vi "Pose3d_Div.vi"(9 "Scalar":dbl, 11 "in Pose3d":T1={"Translation3d"={"X"=0.0, "Y"=0.0, "Z"=0.0}, "Rotation3d"={"Q_quaternion"={"R"=1.0, "V"=[0.0, 0.0, 0.0]}}} {"Translation3d"."Z" format="%14.3f"; "Translation3d"."Y" format="%14.3f"; "Translation3d"."X" format="%14.3f"}) -> (3 "out Pose3d":T1={"Translation3d"={"X"=0.0, "Y"=0.0, "Z"=0.0}, "Rotation3d"={"Q_quaternion"={"R"=1.0, "V"=[0.0, 0.0, 0.0]}}} {"Translation3d"."Z" format="%14.3f"; "Translation3d"."Y" format="%14.3f"; "Translation3d"."X" format="%14.3f"})   [LabVIEW 2019, in "Trajectory_Library.lvlib"]
doc: "Divide the pose by the given scalar and returns the new pose3d. \n\nParameters:\n - IN POSE3D - The input POSE data structure\n - Scalar - The value to divide the pose by.\n\nReturn:\n - OUT POSE3D - The output pose."
uses:
  TypeDef/POSE3D.ctl
  TypeDef/TRANSLATION3D.ctl
  TypeDef/ROTATION3D.ctl
  TypeDef/QUATERNION.ctl
  Translation3d_Create.vi
  Translation3d_GetXYZ.vi
  Rotation3d_Create_AxisAngle.vi
  Rotation3d_GetQuaterion.vi
  Quaternion_Get_Vect.vi
  Quaternion_Get_W.vi
  Quaternion_New.vi
  Rotation3d_Create_Default.vi
  Vector_Norm.vi
  VecBuilder_ArrayBy1Fill.vi
  Quaternion_New_Default.vi
  MatBuilder_Create.vi
  Trajectory_Library.lvlib
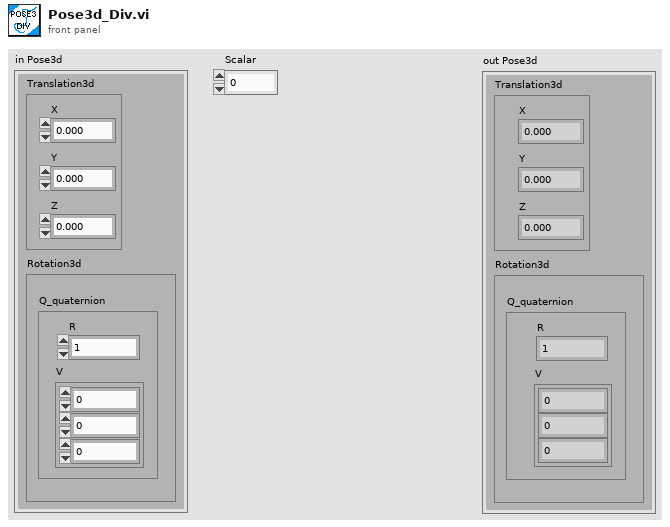
[diagram p1: front panel]
types:
  T1 = typedef "Trajectory_Library.lvlib/POSE3D.ctl" = cluster{"Translation3d":T2, "Rotation3d":T3}
  T2 = typedef "Trajectory_Library.lvlib/TRANSLATION3D.ctl" = cluster{"X":dbl, "Y":dbl, "Z":dbl}
  T3 = typedef "Trajectory_Library.lvlib/ROTATION3D.ctl" = cluster{"Q_quaternion":T4}
  T4 = typedef "Trajectory_Library.lvlib/QUATERNION.ctl" = cluster{"R":dbl, "V":dbl[]}
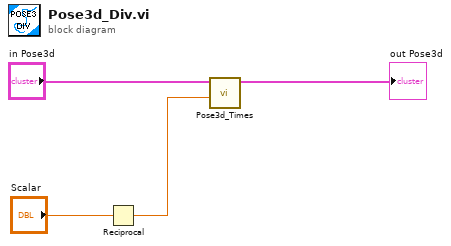
[diagram p0: block diagram]
diagram:
  n1 = Reciprocal(x="Scalar") -> (1/x=w3:dbl)
  n2 = call "Pose3d_Times.vi"("Scalar"=w3, "in Pose3d"="in Pose3d") -> ("out Pose3d"=→"out Pose3d":T1)  [unwired: 9 in]
